vi "Teleop.vi"(10 "Match Info":T1={"Autonomous Elapsed Seconds"=0.0, "TeleOp Elapsed Seconds"=0.0, "Disabled Elapsed Seconds"=0.0, "Visited Autonomous"=FALSE, "Visited TeleOp"=FALSE, "Visited Disabled"=FALSE, "Autonomous Settings"={"Autonomous Style"=enum."Independent", "VI Refnum"=refnum}}, 11 "Call Context":T2) -> ()   [LabVIEW 2016]
doc: "This VI is called for each TeleOp packet received from the DS where the robot is not disabled. It is often used to read from the joysticks and update I/O or to update setpoints for timed control loops. It should complete and return within 20 milliseconds or it may miss DS packets."
uses:
  <vilib>/Rock Robotics/WPI/DriverStation/WPI_DriverStationDerivedRobotMode.ctl
  <vilib>/Rock Robotics/WPI/DriverStation/WPI_DriverStationMatch Info.ctl
  <vilib>/Rock Robotics/WPI/Solenoid/WPI_SolenoidValue.ctl
  <vilib>/Rock Robotics/WPI/Utilities/WPI_GetSetVariantRefNum.vi
  <vilib>/Rock Robotics/Network Tables/NT Write Boolean.vi
  <vilib>/Rock Robotics/WPI/Solenoid/WPI_SolenoidSetEnum.vi
  <vilib>/Rock Robotics/Network Tables/NT Read Boolean.vi
  test2/Robot Global Data.vi
  <vilib>/Rock Robotics/Network Tables/NT Write Number.vi
  <vilib>/Rock Robotics/WPI/RobotDrive/WPI_RobotDriveArcadeDrive_Standard(NoSaturation).vi
  <vilib>/Rock Robotics/Network Tables/NT Write Numeric Array.vi
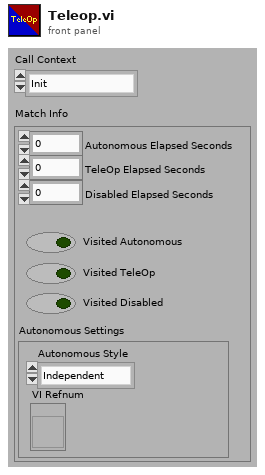
[diagram p1: front panel]
types:
  T1 = typedef "WPI_DriverStationMatch Info.ctl" = cluster{"Autonomous Elapsed Seconds":dbl, "TeleOp Elapsed Seconds":dbl, "Disabled Elapsed Seconds":dbl, "Visited Autonomous":bool, "Visited TeleOp":bool, "Visited Disabled":bool, "Autonomous Settings":cluster{"Autonomous Style":enum16{"Iterative", "Independent"}, "VI Refnum":refnum<vi>}}
  T2 = typedef "WPI_DriverStationDerivedRobotMode.ctl" = enum16{"Init", "Execute", "Stop"}
  T3 = typedef "WPI_SolenoidValue.ctl" = enum16{"Off", "On", "Forward", "Reverse"}
  T4 = typedef "WPI_JoystickDevRef.ctl" = cluster{"Device":T5}
  T5 = typedef "WPI_JoystickDeviceEnum.ctl" = enum16{"USB 0", "USB 1", "USB 2", "USB 3", "USB 4", "USB 5"}
  T6 = cluster{"POVs[0]":i16, "POVs[1]":i16, "POVs[2]":i16, "POVs[3]":i16, "POVs[4]":i16, "POVs[5]":i16, "POVs[6]":i16, "POVs[7]":i16, "POVs[8]":i16}
  T7 = cluster{"Axes[0]":dbl, "Axes[1]":dbl, "Axes[2]":dbl, "Axes[3]":dbl, "Axes[4]":dbl, "Axes[5]":dbl, "Axes[6]":dbl, "Axes[7]":dbl, "Axes[8]":dbl}
  T8 = cluster{"Buttons[0]":bool, "Buttons[1]":bool, "Buttons[2]":bool, "Buttons[3]":bool, "Buttons[4]":bool, "Buttons[5]":bool, "Buttons[6]":bool, "Buttons[7]":bool, "Buttons[8]":bool}
  T9 = typedef "WPI_MotorControlDeviceRef.ctl" = cluster{"DeviceStatus":errorcluster, "Type":T10, "PWM":cluster{"PWM Channel":T11, "DeadBand":T12}, "CAN":cluster{"Device Number":u8, "SetOutput VI Ref":variant, "GetOutput VI Ref":variant, "Enable VI Ref":variant, "Disable VI Ref":variant, "Data":variant}, "Invert":bool}
  T10 = typedef "WPI_MotorControlType.ctl" = enum16{"PWM", "CAN"}
  T11 = typedef "FPGA_DIOPWMChannel.ctl" = enum8{"PWM 0", "PWM 1", "PWM 2", "PWM 3", "PWM 4", "PWM 5", "PWM 6", "PWM 7", "PWM 8", "PWM 9", "PWM MXP 0", "PWM MXP 1", "PWM MXP 2", "PWM MXP 3", "PWM MXP 4", "PWM MXP 5", "PWM MXP 6", "PWM MXP 7", "PWM MXP 8", "PWM MXP 9", "Invalid"}
  T12 = typedef "WPI_PWMDeadband.ctl" = cluster{"Name":string, "maxPositivePwm":i32, "minPositivePwm":i32, "centerPwm":i32, "maxNegativePwm":i32, "minNegativePwm":i32, "angularRange":u16}
  T13 = typedef "WPI_SolenoidDevRef.ctl" = cluster{"DevStatus":errorcluster, "Pneumatics Control Module":u8, "Forward Solenoid Channel":T14, "Reverse Solenoid Channel":T14}
  T14 = typedef "WPI_SolenoidChannel.ctl" = enum8{"Solenoid 0", "Solenoid 1", "Solenoid 2", "Solenoid 3", "Solenoid 4", "Solenoid 5", "Solenoid 6", "Solenoid 7", "Invalid"}
  T15 = typedef "WPI_CompressorDevRef.ctl" = cluster{"DevStatus":errorcluster, "Pneumatics Control Module":u8}
  T16 = typedef "WPI_RobotDriveDevRef.ctl" = cluster{"DevStatus":errorcluster, "Motors[]":T9[], "Square Inputs":bool, "Max Output":dbl}
  T17 = typedef "WPI_GyroDevRef.ctl" = cluster{"DevStatus":errorcluster, "Analog Channel":T18, "Offset":dbl, "Gain (VoltsPerDegree/Second)":dbl, "Gyro Type":enum16{"Analog", "XRS450"}, "Handle":i32, "SPI Bus":T19, "Device Found":bool, "Sample Rate":dbl, "Calibrate On Open":bool}
  T18 = typedef "FPGA_AIChannel.ctl" = enum8{"AI 0", "AI 1", "AI 2", "AI 3", "AI MXP 0", "AI MXP 1", "AI MXP 2", "AI MXP 3", "Invalid"}
  T19 = typedef "spi_bus.ctl" = enum16{"SPI On-Board, CS0", "SPI On-Board, CS1", "SPI On-Board, CS2", "SPI On-Board, CS3", "SPI MXP", "Invalid"}
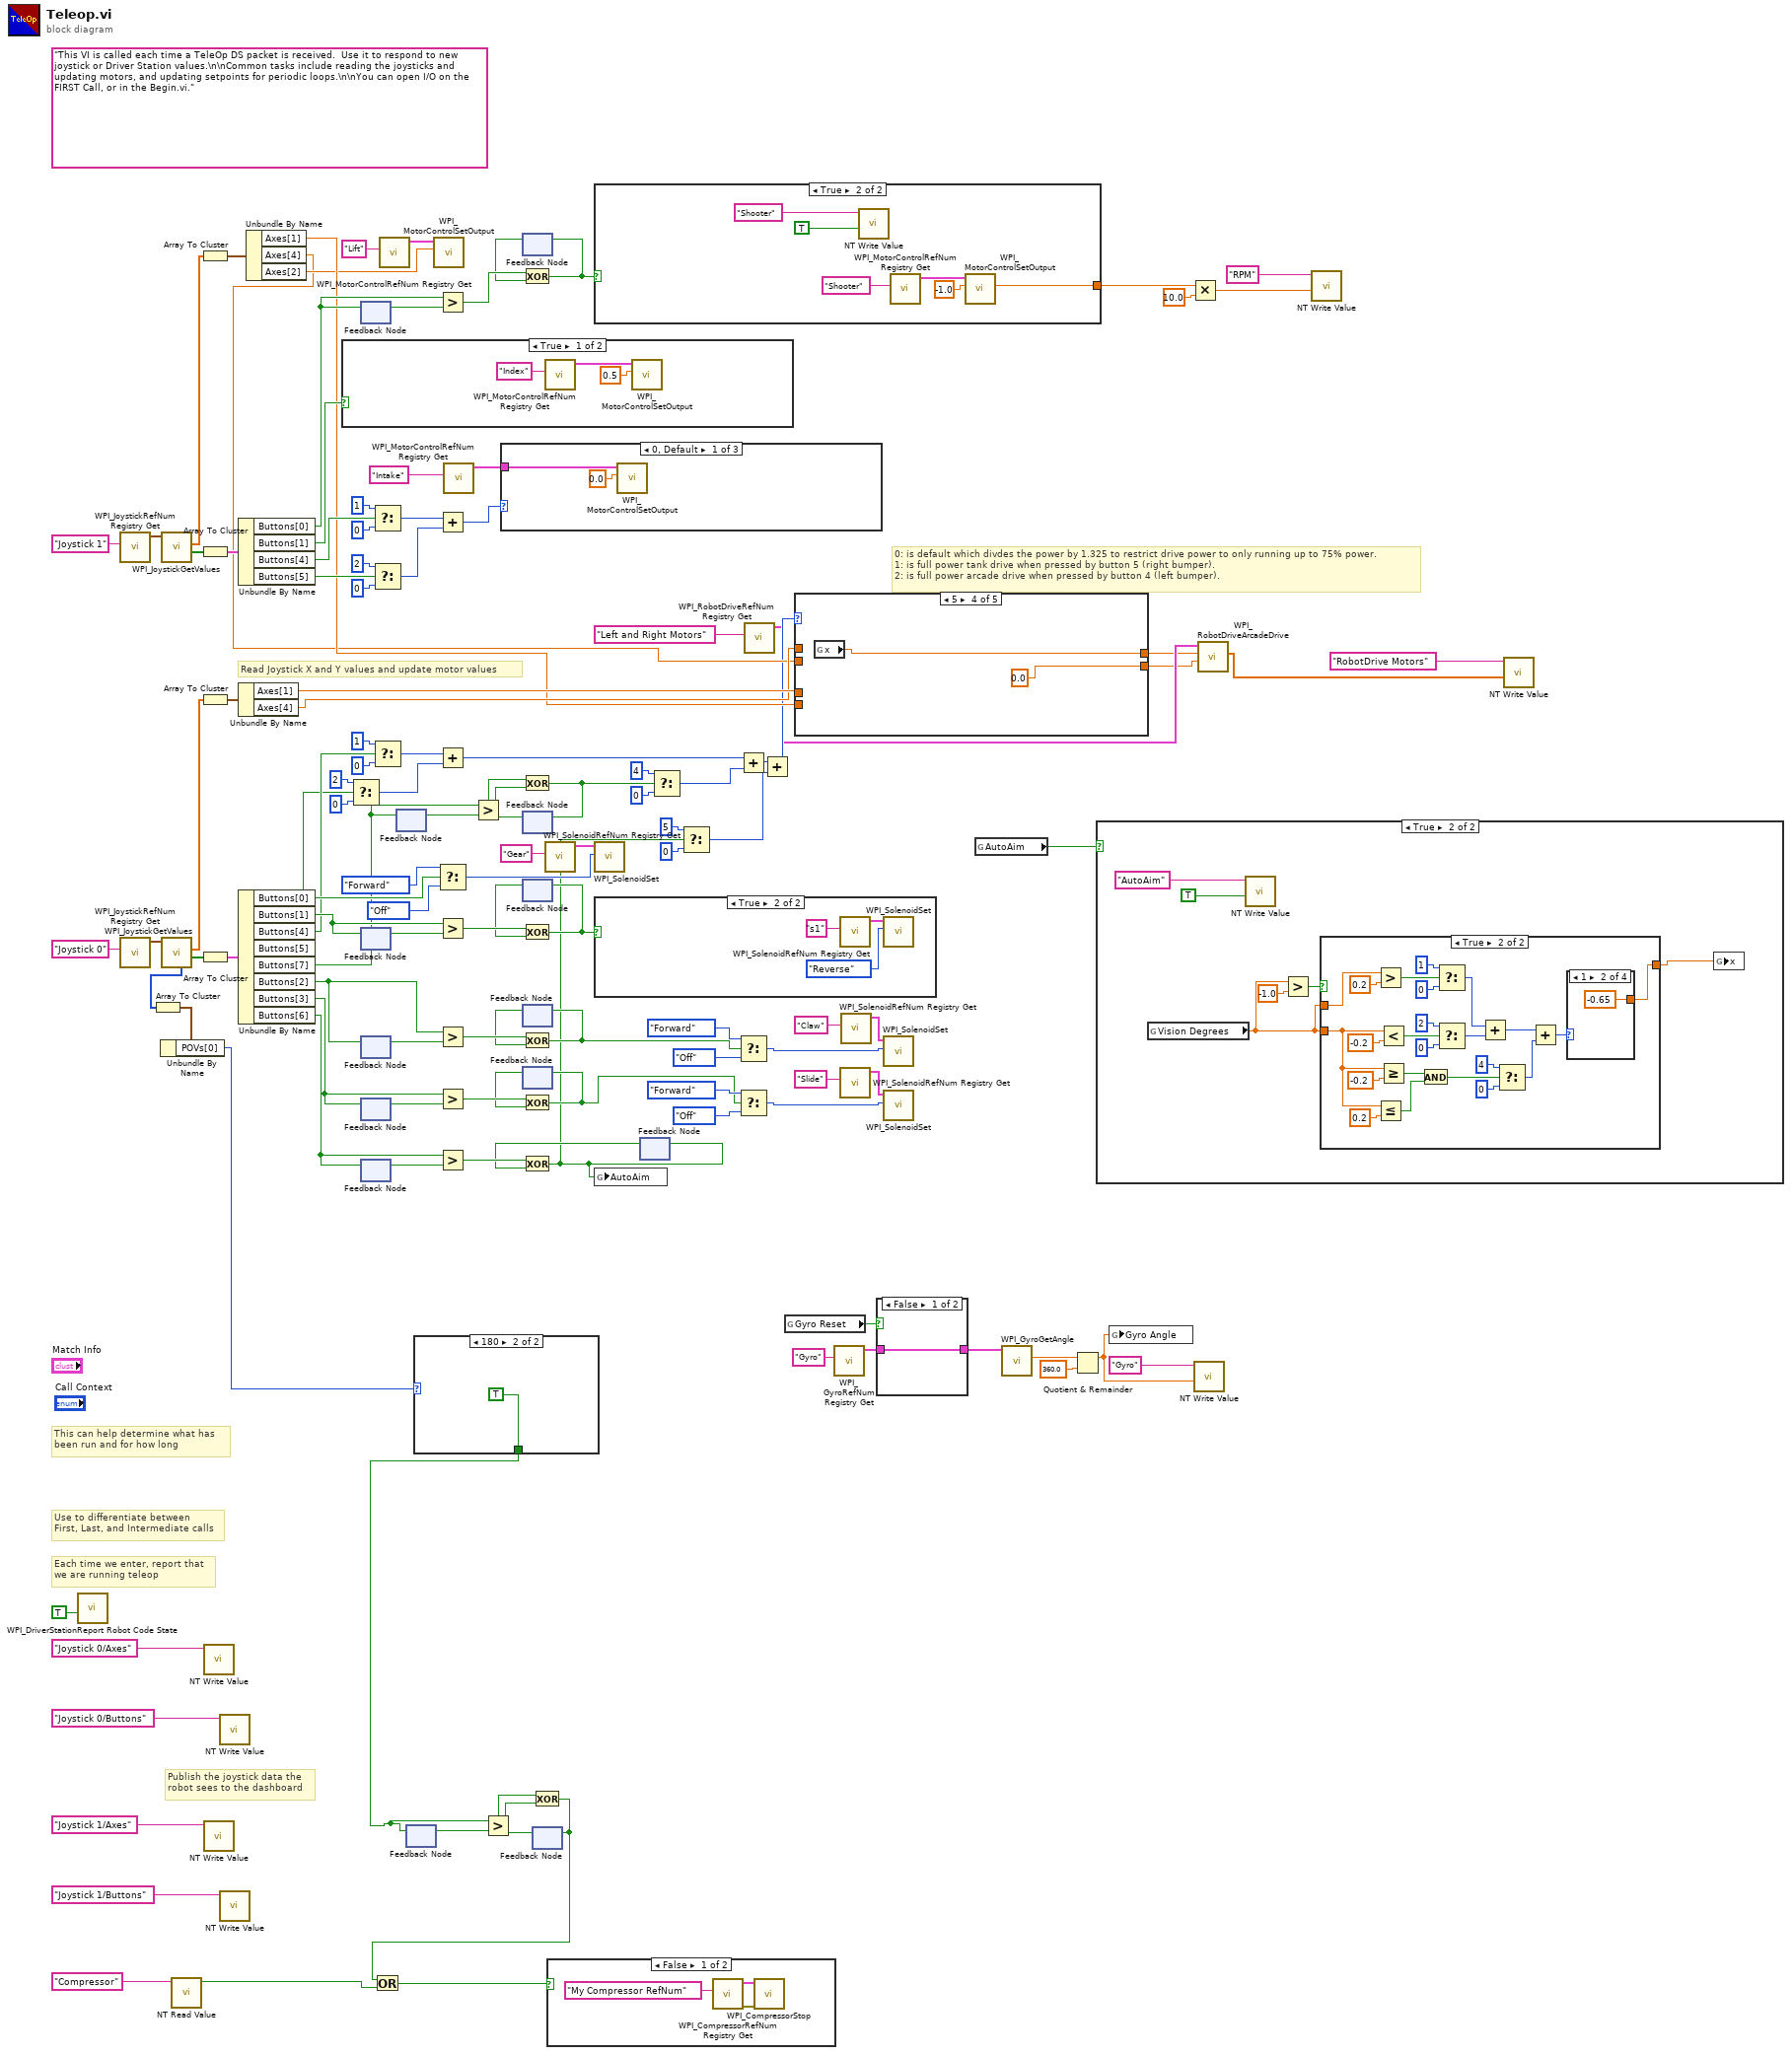
[diagram p0: block diagram]
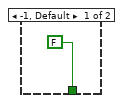
[diagram p2: hidden frame]
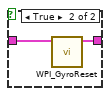
[diagram p3: hidden frame]
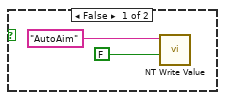
[diagram p4: hidden frame]
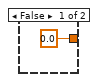
[diagram p5: hidden frame]
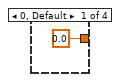
[diagram p6: hidden frame]
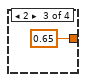
[diagram p7: hidden frame]
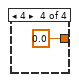
[diagram p8: hidden frame]
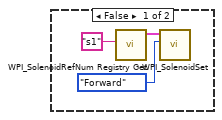
[diagram p9: hidden frame]
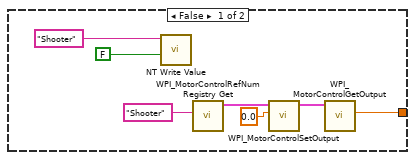
[diagram p10: hidden frame]
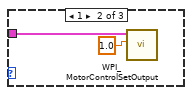
[diagram p11: hidden frame]
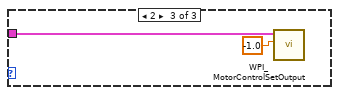
[diagram p12: hidden frame]
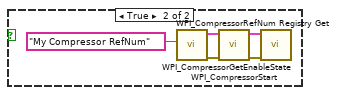
[diagram p13: hidden frame]
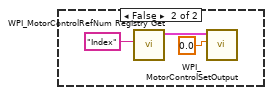
[diagram p14: hidden frame]
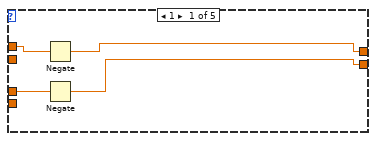
[diagram p15: hidden frame]
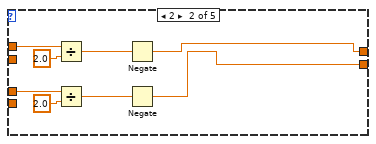
[diagram p16: hidden frame]
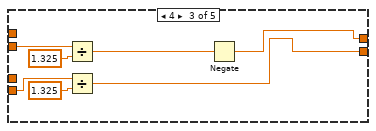
[diagram p17: hidden frame]
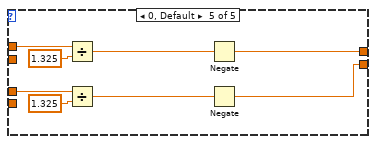
[diagram p18: hidden frame]
diagram:
  (unwired) "This VI is called each time a TeleOp DS packet is received.  Use it to respond to new joystick or Driver Station values.\n\nCommon tasks include reading the joysticks and updating motors, and updating setpoints for periodic loops.\n\nYou can open I/O on the FIRST Call, or in the Begin.vi."
  # "0: is default which divdes the power by 1.325 to restrict drive power to only running up to 75% power.\n1: is full power tank drive when pressed by button 5 (right bumper).\n2: is full power arcade drive when pressed by button 4 (left bumper)."
  # "Publish the joystick data the\nrobot sees to the dashboard"
  # "Each time we enter, report that\nwe are running teleop"
  # "Use to differentiate between\nFirst, Last, and Intermediate calls"
  # "This can help determine what has\nbeen run and for how long"
  # "Read Joystick X and Y values and update motor values"
  n1 = call <vilib>:"WPI_DriverStationReport Robot Code State.vi"("TeleOp"=TRUE ("Autonomous")) -> ()  [unwired: 10 in, 1 out]
  n2 = call <vilib>:"WPI_JoystickRefNum Registry Get.vi"("refnum name"="Joystick 1") -> ("JoystickDevRef"=w101:T4)  [unwired: 1 in, 9 out]
  n3 = call <vilib>:"WPI_JoystickRefNum Registry Get.vi"("refnum name"="Joystick 0") -> ("JoystickDevRef"=w127:T4)  [unwired: 1 in, 9 out]
  n4 = call <vilib>:"WPI_JoystickGetValues.vi"("JoystickDevRef"=w101) -> ("Buttons"=w100:bool[], "Axes"=w70:dbl[])  [unwired: 6 in, 3 out]
  n5 = call <vilib>:"WPI_JoystickGetValues.vi"("JoystickDevRef"=w127) -> ("Buttons"=w118:bool[], "Axes"=w122:dbl[], "POVs"=w9:i16[])  [unwired: 6 in, 2 out]
  n6 = Array To Cluster(array=w9) -> (cluster=w8:T6)
  n7 = Unbundle By Name(w8) -> ("POVs[0]"=w7:i16)
  n8 = call-poly <vilib>:"NT Read Value.vi"("Name"="Compressor") -> ("Boolean"=w10:bool)  [unwired: 9 in, 1 out]
  n9 = Array To Cluster(array=w70) -> (cluster=w69:T7)
  n10 = Array To Cluster(array=w100) -> (cluster=w99:T8)
  n11 = Array To Cluster(array=w122) -> (cluster=w121:T7)
  n12 = Array To Cluster(array=w118) -> (cluster=w117:T8)
  n13 = call-poly <vilib>:"NT Write Value.vi"("Name"="Joystick 0/Axes") -> ()  [unwired: 10 in, 1 out]
  n14 = call-poly <vilib>:"NT Write Value.vi"("Name"="Joystick 1/Axes") -> ()  [unwired: 10 in, 1 out]
  n15 = call-poly <vilib>:"NT Write Value.vi"("Name"="Joystick 0/Buttons") -> ()  [unwired: 10 in, 1 out]
  n16 = call-poly <vilib>:"NT Write Value.vi"("Name"="Joystick 1/Buttons") -> ()  [unwired: 10 in, 1 out]
  n17 = Unbundle By Name(w99) -> ("Buttons[0]"=w68:bool, "Buttons[1]"=w80:bool, "Buttons[4]"=w98:bool, "Buttons[5]"=w97:bool)
  n18 = Unbundle By Name(w121) -> ("Axes[1]"=w120:dbl, "Axes[4]"=w119:dbl)
  n19 = Unbundle By Name(w117) -> ("Buttons[0]"=w79:bool, "Buttons[1]"=w87:bool, "Buttons[4]"=w72:bool, "Buttons[5]"=w71:bool, "Buttons[7]"=w54:bool, "Buttons[2]"=w50:bool, "Buttons[3]"=w34:bool, "Buttons[6]"=w30:bool)
  n20 = Unbundle By Name(w69) -> ("Axes[1]"=w59:dbl, "Axes[4]"=w57:dbl, "Axes[2]"=w58:dbl)
  n21 = case shown="True" w80 {
    frame True {
      n22 = call <vilib>:"WPI_MotorControlRefNum Registry Get.vi"("refnum name"="Index") -> ("MotorControlDevRef"=w131:T9)  [unwired: 9 in, 1 out]
      n23 = call <vilib>:"WPI_MotorControlSetOutput.vi"("Output"=0.5, "MotorControlDevRef"=w131) -> ()  [unwired: 7 in, 3 out]
    }
    frame False {
      n24 = call <vilib>:"WPI_MotorControlRefNum Registry Get.vi"("refnum name"="Index") -> ("MotorControlDevRef"=w134:T9)  [unwired: 9 in, 1 out]
      n25 = call <vilib>:"WPI_MotorControlSetOutput.vi"("Output"=0.0, "MotorControlDevRef"=w134) -> ()  [unwired: 7 in, 3 out]
    }
  }
  n26 = Select(t=2 ("f"), s=w71, f=0) -> (s? t:f=w73:i32)
  n27 = feedback #1() -> (w83:bool)  [unwired: 1 in]
  n28 = feedback-in #1(w68) -> ()
  n29 = feedback #2() -> (w106:bool)  [unwired: 1 in]
  n30 = feedback-in #2(w87) -> ()
  n31 = feedback #3() -> (w53:bool)  [unwired: 1 in]
  n32 = feedback-in #3(w50) -> ()
  n33 = feedback #4() -> (w49:bool)  [unwired: 1 in]
  n34 = feedback-in #4(w34) -> ()
  n35 = feedback #5() -> (w33:bool)  [unwired: 1 in]
  n36 = feedback-in #5(w30) -> ()
  n37 = Select(t=1, s=w98, f=0) -> (s? t:f=w92:i32)
  n38 = Select(t=2 ("f"), s=w97, f=0) -> (s? t:f=w91:i32)
  n39 = Select(t=1, s=w72, f=0) -> (s? t:f=w74:i32)
  n40 = call <vilib>:"WPI_MotorControlRefNum Registry Get.vi"("refnum name"="Lift") -> ("MotorControlDevRef"=w115:T9)  [unwired: 9 in, 1 out]
  n41 = feedback #6() -> (w67:bool)  [unwired: 1 in]
  n42 = feedback-in #6(w54) -> ()
  n43 = feedback #7() -> (w5:bool)  [unwired: 1 in]
  n44 = case shown="180" w7 {
    tunnel: [FALSE TRUE] -> w2
    frame -1, Default {
    }
    frame 180 {
    }
  }
  n45 = feedback-in #7(w2) -> ()
  n46 = call <vilib>:"WPI_MotorControlSetOutput.vi"("Output"=w58, "MotorControlDevRef"=w115) -> ()  [unwired: 7 in, 3 out]
  n47 = Greater?(x=w68, y=w83) -> (0:w82:bool)
  n48 = Add(x=w92, y=w91) -> (x+y=w90:i32)
  n49 = Add(x=w74, y=w73) -> (x+y=w60:i32)
  n50 = Select(t=WPI_SolenoidValue."Forward" ("Value"), s=w79, f=WPI_SolenoidValue."Off" ("Value")) -> (s? t:f=w107:T3)
  n51 = Greater?(x=w87, y=w106) -> (0:w105:bool)
  n52 = Greater?(x=w50, y=w53) -> (0:w52:bool)
  n53 = Greater?(x=w34, y=w49) -> (0:w48:bool)
  n54 = Greater?(x=w30, y=w33) -> (0:w32:bool)
  n55 = call <vilib>:"WPI_MotorControlRefNum Registry Get.vi"("refnum name"="Intake") -> ("MotorControlDevRef"=w109:T9)  [unwired: 9 in, 1 out]
  n56 = Greater?(x=w54, y=w67) -> (0:w66:bool)
  n57 = Greater?(x=w2, y=w5) -> (0:w4:bool)
  n58 = case shown="0, Default" w90 {
    tunnel: w109 -> [w139 w141 w142]
    frame 0, Default {
      n59 = call <vilib>:"WPI_MotorControlSetOutput.vi"("Output"=0.0, "MotorControlDevRef"=w139) -> ()  [unwired: 7 in, 3 out]
    }
    frame 1 {
      n60 = call <vilib>:"WPI_MotorControlSetOutput.vi"("Output"=1.0, "MotorControlDevRef"=w141) -> ()  [unwired: 7 in, 3 out]
    }
    frame 2 {
      n61 = call <vilib>:"WPI_MotorControlSetOutput.vi"("Output"=-1.0, "MotorControlDevRef"=w142) -> ()  [unwired: 7 in, 3 out]
    }
  }
  n62 = feedback #8() -> (w81:bool)  [unwired: 1 in]
  n63 = Exclusive Or(1:w81, 2:w82) -> (0:w55:bool)
  n64 = feedback-in #8(w55) -> ()
  n65 = feedback #9() -> (w65:bool)  [unwired: 1 in]
  n66 = Exclusive Or(1:w65, 2:w66) -> (0:w62:bool)
  n67 = feedback-in #9(w62) -> ()
  n68 = feedback #10() -> (w104:bool)  [unwired: 1 in]
  n69 = Exclusive Or(1:w104, 2:w105) -> (0:w103:bool)
  n70 = feedback-in #10(w103) -> ()
  n71 = feedback #11() -> (w51:bool)  [unwired: 1 in]
  n72 = Exclusive Or(1:w51, 2:w52) -> (0:w35:bool)
  n73 = feedback-in #11(w35) -> ()
  n74 = feedback #12() -> (w47:bool)  [unwired: 1 in]
  n75 = Exclusive Or(1:w47, 2:w48) -> (0:w41:bool)
  n76 = feedback-in #12(w41) -> ()
  n77 = feedback #13() -> (w3:bool)  [unwired: 1 in]
  n78 = Exclusive Or(1:w3, 2:w4) -> (0:w1:bool)
  n79 = Or(x=w1, y=w10) -> (x .or. y?=w6:bool)
  n80 = feedback-in #13(w1) -> ()
  n81 = call <vilib>:"WPI_SolenoidRefNum Registry Get.vi"("refnum name"="Gear") -> ("SolenoidDevRef"=w112:T13)  [unwired: 9 in, 1 out]
  n82 = case shown="False" w6 {
    frame False {
      n83 = call <vilib>:"WPI_CompressorRefNum Registry Get.vi"("refnum name"="My Compressor RefNum") -> ("error out"=w145:errorcluster, "CompressorDevRef"=w146:T15)  [unwired: 9 in]
      n84 = call <vilib>:"WPI_CompressorStop.vi"("error in (no error)"=w145, "CompressorDevRef"=w146) -> ()  [unwired: 8 in, 2 out]
    }
    frame True {
      n85 = call <vilib>:"WPI_CompressorRefNum Registry Get.vi"("refnum name"="My Compressor RefNum") -> ("error out"=w149:errorcluster, "CompressorDevRef"=w150:T15)  [unwired: 9 in]
      n86 = call <vilib>:"WPI_CompressorStart.vi"("error in (no error)"=w149, "CompressorDevRef"=w150) -> ("error out"=w147:errorcluster, "CompressorDevRef"=w148:T15)  [unwired: 8 in]
      n87 = call <vilib>:"WPI_CompressorGetEnableState.vi"("error in (no error)"=w147, "CompressorDevRef"=w148) -> ()  [unwired: 6 in, 4 out]
    }
  }
  n88 = case shown="True" w55 {
    tunnel: [w154 w160] -> w56
    frame False {
      n89 = call-poly <vilib>:"NT Write Value.vi"("Boolean"=FALSE, "Name"="Shooter") -> ()  [unwired: 9 in, 1 out]
      n90 = call <vilib>:"WPI_MotorControlRefNum Registry Get.vi"("refnum name"="Shooter") -> ("MotorControlDevRef"=w157:T9)  [unwired: 9 in, 1 out]
      n91 = call <vilib>:"WPI_MotorControlSetOutput.vi"("Output"=0.0, "MotorControlDevRef"=w157) -> ("MotorControlDevRef"=w155:T9)  [unwired: 7 in, 2 out]
      n92 = call <vilib>:"WPI_MotorControlGetOutput.vi"("MotorControlDevRef"=w155) -> ("Output"=w154:dbl)  [unwired: 8 in, 2 out]
    }
    frame True {
      n93 = call-poly <vilib>:"NT Write Value.vi"("Boolean"=TRUE, "Name"="Shooter") -> ()  [unwired: 9 in, 1 out]
      n94 = call <vilib>:"WPI_MotorControlRefNum Registry Get.vi"("refnum name"="Shooter") -> ("MotorControlDevRef"=w163:T9)  [unwired: 9 in, 1 out]
      n95 = call <vilib>:"WPI_MotorControlSetOutput.vi"("Output"=-1.0, "MotorControlDevRef"=w163) -> ("Motor Output"=w160:dbl)  [unwired: 7 in, 2 out]
    }
  }
  n96 = call-poly <vilib>:"WPI_SolenoidSet.vi"("Value"=w107, "SolenoidDevRef"=w112) -> ()  [unwired: 1 in, 9 out]
  n97 = case shown="True" w103 {
    frame False {
      n98 = call <vilib>:"WPI_SolenoidRefNum Registry Get.vi"("refnum name"="s1") -> ("SolenoidDevRef"=w167:T13)  [unwired: 9 in, 1 out]
      n99 = call-poly <vilib>:"WPI_SolenoidSet.vi"("Value"=WPI_SolenoidValue."Forward", "SolenoidDevRef"=w167) -> ()  [unwired: 1 in, 9 out]
    }
    frame True {
      n100 = call <vilib>:"WPI_SolenoidRefNum Registry Get.vi"("refnum name"="s1") -> ("SolenoidDevRef"=w170:T13)  [unwired: 9 in, 1 out]
      n101 = call-poly <vilib>:"WPI_SolenoidSet.vi"("Value"=WPI_SolenoidValue."Reverse", "SolenoidDevRef"=w170) -> ()  [unwired: 1 in, 9 out]
    }
  }
  n102 = feedback #14() -> (w31:bool)  [unwired: 1 in]
  n103 = Exclusive Or(1:w31, 2:w32) -> (0:w24:bool)
  n104 = global write "Robot Global Data.vi" "AutoAim"(w24) -> ()
  n105 = feedback-in #14(w24) -> ()
  n106 = Select(t=4, s=w62, f=0) -> (s? t:f=w61:i32)
  n107 = Select(t=5, s=w24, f=0) -> (s? t:f=w25:i32)
  n108 = Add(x=w60, y=w61) -> (x+y=w26:i32)
  n109 = Select(t=WPI_SolenoidValue."Forward" ("Value"), s=w35, f=WPI_SolenoidValue."Off" ("Value")) -> (s? t:f=w36:T3)
  n110 = Select(t=WPI_SolenoidValue."Forward" ("Value"), s=w41, f=WPI_SolenoidValue."Off" ("Value")) -> (s? t:f=w42:T3)
  n111 = call <vilib>:"WPI_RobotDriveRefNum Registry Get.vi"("refnum name"="Left and Right Motors") -> ("RobotDriveDevRef"=w22:T16)  [unwired: 1 in, 9 out]
  n112 = Add(x=w26, y=w25) -> (x+y=w27:i32)
  n113 = global read "Robot Global Data.vi" "Gyro Reset"() -> (w15:bool)
  n114 = case shown="5" w27 {
    tunnel: w120 -> [w173 w182 _ _ w199]
    tunnel: w119 -> [w174 w179 _ _ w197]
    tunnel: w59 -> [_ _ w188 _ _]
    tunnel: w57 -> [_ _ w186 _ _]
    tunnel: [w172 w176 w184 w191 w193] -> w20
    tunnel: [w171 w175 w183 0.0 w192] -> w19
    frame 1 {
      n115 = Negate(x=w174) -> (-x=w172:dbl)
      n116 = Negate(x=w173) -> (-x=w171:dbl)
    }
    frame 2 {
      n117 = Divide(x=w179, y=2.0) -> (x/y=w178:dbl)
      n118 = Divide(x=w182, y=2.0) -> (x/y=w177:dbl)
      n119 = Negate(x=w178) -> (-x=w176:dbl)
      n120 = Negate(x=w177) -> (-x=w175:dbl)
    }
    frame 4 {
      n121 = Divide(x=w186, y=1.325) -> (x/y=w185:dbl)
      n122 = Divide(x=w188, y=1.325) -> (x/y=w183:dbl)
      n123 = Negate(x=w185) -> (-x=w184:dbl)
    }
    frame 5 {
      n124 = global read "Robot Global Data.vi" "x"() -> (w191:dbl)
    }
    frame 0, Default {
      n125 = Divide(x=w197, y=1.325) -> (x/y=w194:dbl)
      n126 = Divide(x=w199, y=1.325) -> (x/y=w198:dbl)
      n127 = Negate(x=w194) -> (-x=w193:dbl)
      n128 = Negate(x=w198) -> (-x=w192:dbl)
    }
  }
  n129 = call <vilib>:"WPI_GyroRefNum Registry Get.vi"("refnum name"="Gyro") -> ("GyroDevRef"=w14:T17)  [unwired: 9 in, 1 out]
  n130 = call <vilib>:"WPI_SolenoidRefNum Registry Get.vi"("refnum name"="Slide") -> ("SolenoidDevRef"=w44:T13)  [unwired: 9 in, 1 out]
  n131 = call <vilib>:"WPI_SolenoidRefNum Registry Get.vi"("refnum name"="Claw") -> ("SolenoidDevRef"=w38:T13)  [unwired: 9 in, 1 out]
  n132 = case shown="False" w15 {
    tunnel: w14 -> [w200 w202]
    tunnel: [w200 w201] -> w13
    frame False {
    }
    frame True {
      n133 = call <vilib>:"WPI_GyroReset.vi"("GyroDevRef"=w202) -> ("GyroDevRef"=w201:T17)  [unwired: 9 in, 1 out]
    }
  }
  n134 = call-poly <vilib>:"WPI_SolenoidSet.vi"("Value"=w36, "SolenoidDevRef"=w38) -> ()  [unwired: 1 in, 9 out]
  n135 = call-poly <vilib>:"WPI_SolenoidSet.vi"("Value"=w42, "SolenoidDevRef"=w44) -> ()  [unwired: 1 in, 9 out]
  n136 = global read "Robot Global Data.vi" "AutoAim"() -> (w23:bool)
  n137 = call <vilib>:"WPI_GyroGetAngle.vi"("GyroDevRef"=w13) -> ("Angle"=w18:dbl)  [unwired: 6 in, 4 out]
  n138 = Quotient & Remainder(x=w18, y=360.0) -> (x-y*floor(x/y)=w12:dbl)  [unwired: 1 out]
  n139 = case shown="True" w23 {
    frame False {
      n140 = call-poly <vilib>:"NT Write Value.vi"("Boolean"=FALSE, "Name"="AutoAim") -> ()  [unwired: 9 in, 1 out]
    }
    frame True {
      n141 = global read "Robot Global Data.vi" "Vision Degrees"() -> (w206:dbl)
      n142 = call-poly <vilib>:"NT Write Value.vi"("Boolean"=TRUE, "Name"="AutoAim") -> ()  [unwired: 9 in, 1 out]
      n143 = Greater?(x=w206, y=-1.0) -> (0:w207:bool)
      n144 = case shown="True" w207 {
        tunnel: [0.0 w224] -> w205
        tunnel: w206 -> [_ w223]
        tunnel: w206 -> [_ w221]
        frame False {
        }
        frame True {
          n145 = Greater?(x=w223, y=0.2) -> (0:w232:bool)
          n146 = Less Or Equal?(x=w221, y=0.2) -> (x <= y?=w219:bool)
          n147 = Less?(x=w221, y=-0.2) -> (x < y?=w231:bool)
          n148 = Greater Or Equal?(x=w221, y=-0.2) -> (x >= y?=w218:bool)
          n149 = And(x=w218, y=w219) -> (x .and. y?=w217:bool)
          n150 = Select(t=1, s=w232, f=0) -> (s? t:f=w226:i32)
          n151 = Select(t=2 ("f"), s=w231, f=0) -> (s? t:f=w225:i32)
          n152 = Add(x=w226, y=w225) -> (x+y=w214:i32)
          n153 = Select(t=4, s=w217, f=0) -> (s? t:f=w213:i32)
          n154 = Add(x=w214, y=w213) -> (x+y=w212:i32)
          n155 = case shown="1" w212 {
            tunnel: [0.0 ("Y axis value") -0.65 ("X axis value") 0.65 ("X axis value") 0.0] -> w224
            frame 0, Default {
            }
            frame 1 {
            }
            frame 2 {
            }
            frame 4 {
            }
          }
        }
      }
      n156 = global write "Robot Global Data.vi" "x"(w205) -> ()
    }
  }
  n157 = global write "Robot Global Data.vi" "Gyro Angle"(w12) -> ()
  n158 = Multiply(x=w56, y=10.0) -> (x*y=w85:dbl)
  n159 = call-poly <vilib>:"NT Write Value.vi"("Numeric"=w12, "Name"="Gyro") -> ()  [unwired: 9 in, 1 out]
  n160 = call-poly <vilib>:"WPI_RobotDriveArcadeDrive.vi"("Y axis value"=w19, "X axis value"=w20, "RobotDriveDevRef"=w22) -> ("Motor Values"=w21:dbl[])  [unwired: 6 in, 2 out]
  n161 = call-poly <vilib>:"NT Write Value.vi"("Numeric"=w85, "Name"="RPM") -> ()  [unwired: 9 in, 1 out]
  n162 = call-poly <vilib>:"NT Write Value.vi"("Numeric Array"=w21, "Name"="RobotDrive Motors") -> ()  [unwired: 9 in, 1 out]
